vi "Read MXN_.vi"(8 "error in (no error)":errorcluster, 11 "Soda_Actor in":refnum<class "Soda_Actor.lvclass">) -> (0 "error out":errorcluster, 2 "MXN?":bool, 3 "Soda_Actor out":refnum<class "Soda_Actor.lvclass">)   [LabVIEW 2019, in "Soda_Actor.lvlib" / "Soda_Actor.lvclass"]
uses:
  Soda_Actor.lvclass
  Soda_Actor.lvclass/Soda_Actor.ctl
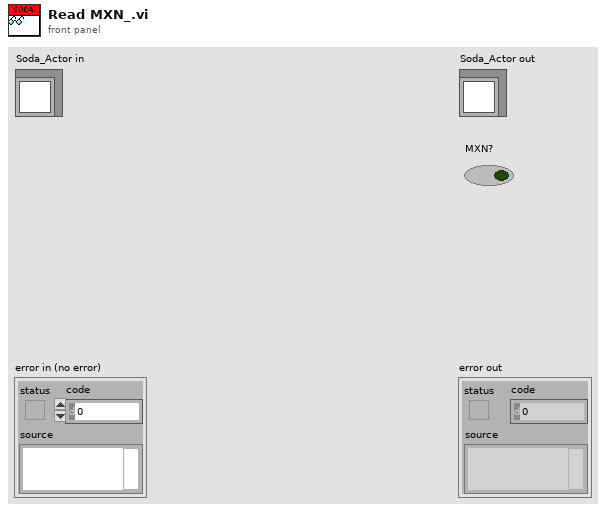
[diagram p1: front panel]
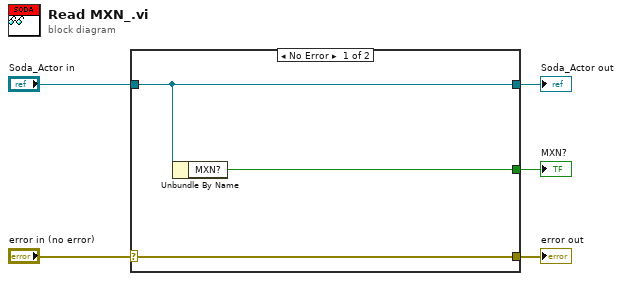
[diagram p0: block diagram]
diagram:
  n1 = case shown="No Error" "error in (no error)" {
    selector: "error in (no error)" -> [w8 w9]
    tunnel: [w8 w9] -> w4
    tunnel: [w7 w10] -> w2
    tunnel: "Soda_Actor in" -> [w7 w10]
    tunnel: [w6 _] -> w1
    frame No Error {
      n2 = Unbundle By Name(w7) -> ("MXN?"=w6:bool)
    }
    frame Error {
    }
  }
  "error out" <- w4
  "Soda_Actor out" <- w2
  "MXN?" <- w1
